vi "Construct.vi"(8 "error in (no error)":errorcluster, 11 "gRPCid":T1) -> (0 "error out":errorcluster, 3 "GRPCMessage out":refnum<class "GRPCMessage.lvclass">)   [LabVIEW 2019, in "MicronGRPCServer.lvlib" / "GRPCMessage.lvclass"]
uses:
  GRPCMessage.lvclass
  <vilib>/gRPC/LabVIEW gRPC Library/Shared/grpcId.ctl
  GRPCMessage.lvclass/GRPCMessage.ctl
  <vilib>/gRPC/LabVIEW gRPC Library/grpc-lvsupport-release.lvlib
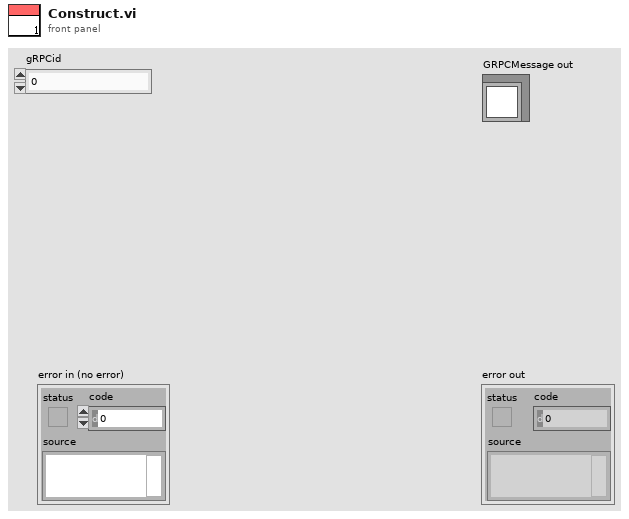
[diagram p1: front panel]
types:
  T1 = typedef "grpc-lvsupport-release.lvlib/grpcId.ctl" = u64
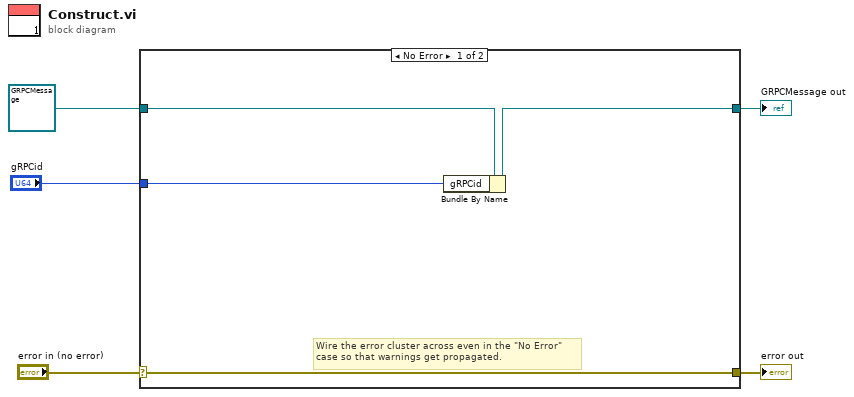
[diagram p0: block diagram]
diagram:
  n1 = case shown="No Error" "error in (no error)" {
    selector: "error in (no error)" -> [w8 w11]
    tunnel: [w8 w11] -> w4
    tunnel: [w7 w10] -> w2
    tunnel: refnum<class "GRPCMessage.lvclass"> refnum ("GRPCMessage in") -> [w9 w10]
    tunnel: "gRPCid" -> [w6 _]
    frame No Error {
      # "Wire the error cluster across even in the \"No Error\"\ncase so that warnings get propagated."
      n2 = Bundle By Name(cluster=w9, "gRPCid"=w6) -> (w7:refnum<class "GRPCMessage.lvclass">)
    }
    frame Error {
    }
  }
  "error out" <- w4
  "GRPCMessage out" <- w2
